vi "DriveBegin.vi"(8 "error in (no error)":errorcluster) -> (0 "error out":errorcluster)   [LabVIEW 2020]
doc: "Begin for Drive\n\nInputs:\n -- Error in -- Error cluster -- propagated error input\n\nOutputs:\n -- Error out -- Error cluster -- progated error output"
uses:
  <vilib>/Rock Robotics/SystemInterfaces/DIO/FPGA_DIOPWMChannel.ctl
  DriveGlobal.vi
  <vilib>/Rock Robotics/WPI/ThirdParty/JAS_Junk/TrajLib/Trajectory_Library.lvlib
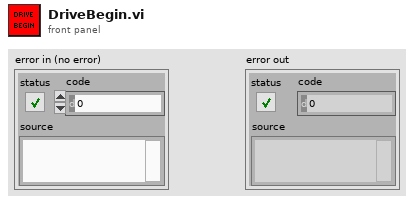
[diagram p1: front panel]
types:
  T1 = typedef "FPGA_DIOPWMChannel.ctl" = enum8{"PWM 0", "PWM 1", "PWM 2", "PWM 3", "PWM 4", "PWM 5", "PWM 6", "PWM 7", "PWM 8", "PWM 9", "PWM MXP 0", "PWM MXP 1", "PWM MXP 2", "PWM MXP 3", "PWM MXP 4", "PWM MXP 5", "PWM MXP 6", "PWM MXP 7", "PWM MXP 8", "PWM MXP 9", "Invalid"}
  T2 = typedef "Trajectory_Library.lvlib/TRANSLATION2D.ctl" = cluster{"X":dbl, "Y":dbl}
  T3 = typedef "Trajectory_Library.lvlib/SWERVE_DRIVE_KINEMATICS.ctl" = cluster{"NumModules":i32, "InverseKinematics":T4, "ForwardKinematics":T4, "Modules":T2[], "PrevCoR":T2, "SavedModuleStates":T5[]}
  T4 = typedef "NI_Matrix.lvlib/RealMatrix.ctl" = dbl[][]
  T5 = typedef "Trajectory_Library.lvlib/SWERVE_DRIVE_MODULE_STATE.ctl" = cluster{"Speed":dbl, "Angle":T6}
  T6 = typedef "Trajectory_Library.lvlib/ROTATION2D.ctl" = cluster{"VALUE":dbl, "COS":dbl, "SIN":dbl}
  T7 = typedef "WPI_PWMDeviceRef.ctl" = cluster{"DeviceStatus":errorcluster, "PWM Channel":T1}
  T8 = typedef "ADIS16470 Device Reference.ctl" = cluster{"DevStatus":errorcluster, "Hardware Config":T9, "Calibration Complete":refnum<notifier>, "Status Reference":refnum<data-value>, "Data Reference":refnum<data-value>, "Sychronous Process VI":T13, "Cmd FIFO":refnum<k33>, "Source":T14, "Data FIFO":refnum<k33>, "Calibration Time (ms)":u32, "Data Reference":refnum<data-value>}
  T9 = typedef "ADIS16470 Hardware Configuration.ctl" = cluster{"SPI Clock Rate (Hz)":dbl, "IMU SPI Mode (3)":T10, "IMU Reset Pin":T11, "IMU SPI Bus":T12, "IMU Data Ready Pin":T11, "Stall Config":cluster{"Pow2BytesPerRead":u8, "StallTicks":u16, "CsToSclkTicks":u8}}
  T10 = typedef "WPI_SPIMode.ctl" = enum16{"Mode 0 (Clk Idle Low,Sample on Leading)", "Mode 1 (Clk Idle Low,Sample on Trailing)", "Mode 2 (Clk Idle High,Sample on Leading)", "Mode 3 (Clk Idle High,Sample on Trailing)"}
  T11 = typedef "FPGA_DIOChannel.ctl" = enum8{"DIO 0", "DIO 1", "DIO 2", "DIO 3", "DIO 4", "DIO 5", "DIO 6", "DIO 7", "DIO 8", "DIO 9", "DIO MXP 0", "DIO MXP 1", "DIO MXP 2", "DIO MXP 3", "DIO MXP 4", "DIO MXP 5", "DIO MXP 6", "DIO MXP 7", "DIO MXP 8", "DIO MXP 9", "DIO MXP 10", "DIO MXP 11", "DIO MXP 12", "DIO MXP 13", "DIO MXP 14", "DIO MXP 15", "SPI Port CS1", "SPI Port CS2", "SPI Port CS3", "SPI Port MISO", "SPI Port MOSI", "Invalid"}
  T12 = typedef "spi_bus.ctl" = enum16{"SPI On-Board, CS0", "SPI On-Board, CS1", "SPI On-Board, CS2", "SPI On-Board, CS3", "SPI MXP", "Invalid"}
  T13 = typedef "ADIS16470 Process.ctl" = refnum<vi>
  T14 = typedef "FPGA_CounterEncoderSourceConvertionLVSourceType.ctl" = cluster{"DevStatus":errorcluster, "AnalogTriggerMode?":bool, "DigitalMode":cluster{"DIO Channel":T15}, "AnalogTriggerMode":cluster{"AnalogTriggerIndex":T16, "OutputType":T17}}
  T15 = typedef "FPGA_DIODigitalSourceChannel.ctl" = enum8{"DIO 0", "DIO 1", "DIO 2", "DIO 3", "DIO 4", "DIO 5", "DIO 6", "DIO 7", "DIO 8", "DIO 9", "DIO MXP 0", "DIO MXP 1", "DIO MXP 2", "DIO MXP 3", "DIO MXP 4", "DIO MXP 5", "DIO MXP 6", "DIO MXP 7", "DIO MXP 8", "DIO MXP 9", "DIO MXP 10", "DIO MXP 11", "DIO MXP 12", "DIO MXP 13", "DIO MXP 14", "DIO MXP 15", "SPI Port CS1", "SPI Port CS2", "SPI Port CS3", "SPI Port MISO", "SPI Port MOSI", "Disabled"}
  T16 = typedef "FPGA_AnalogTriggerIndex.ctl" = enum8{"Trig 0", "Trig 1", "Trig 2", "Trig 3", "Trig 4", "Trig 5", "Trig 6", "Trig 7", "Invalid"}
  T17 = typedef "FPGA_AnalogTriggerOutType.ctl" = enum16{"InWindow", "TriggerState", "Rising", "Falling"}
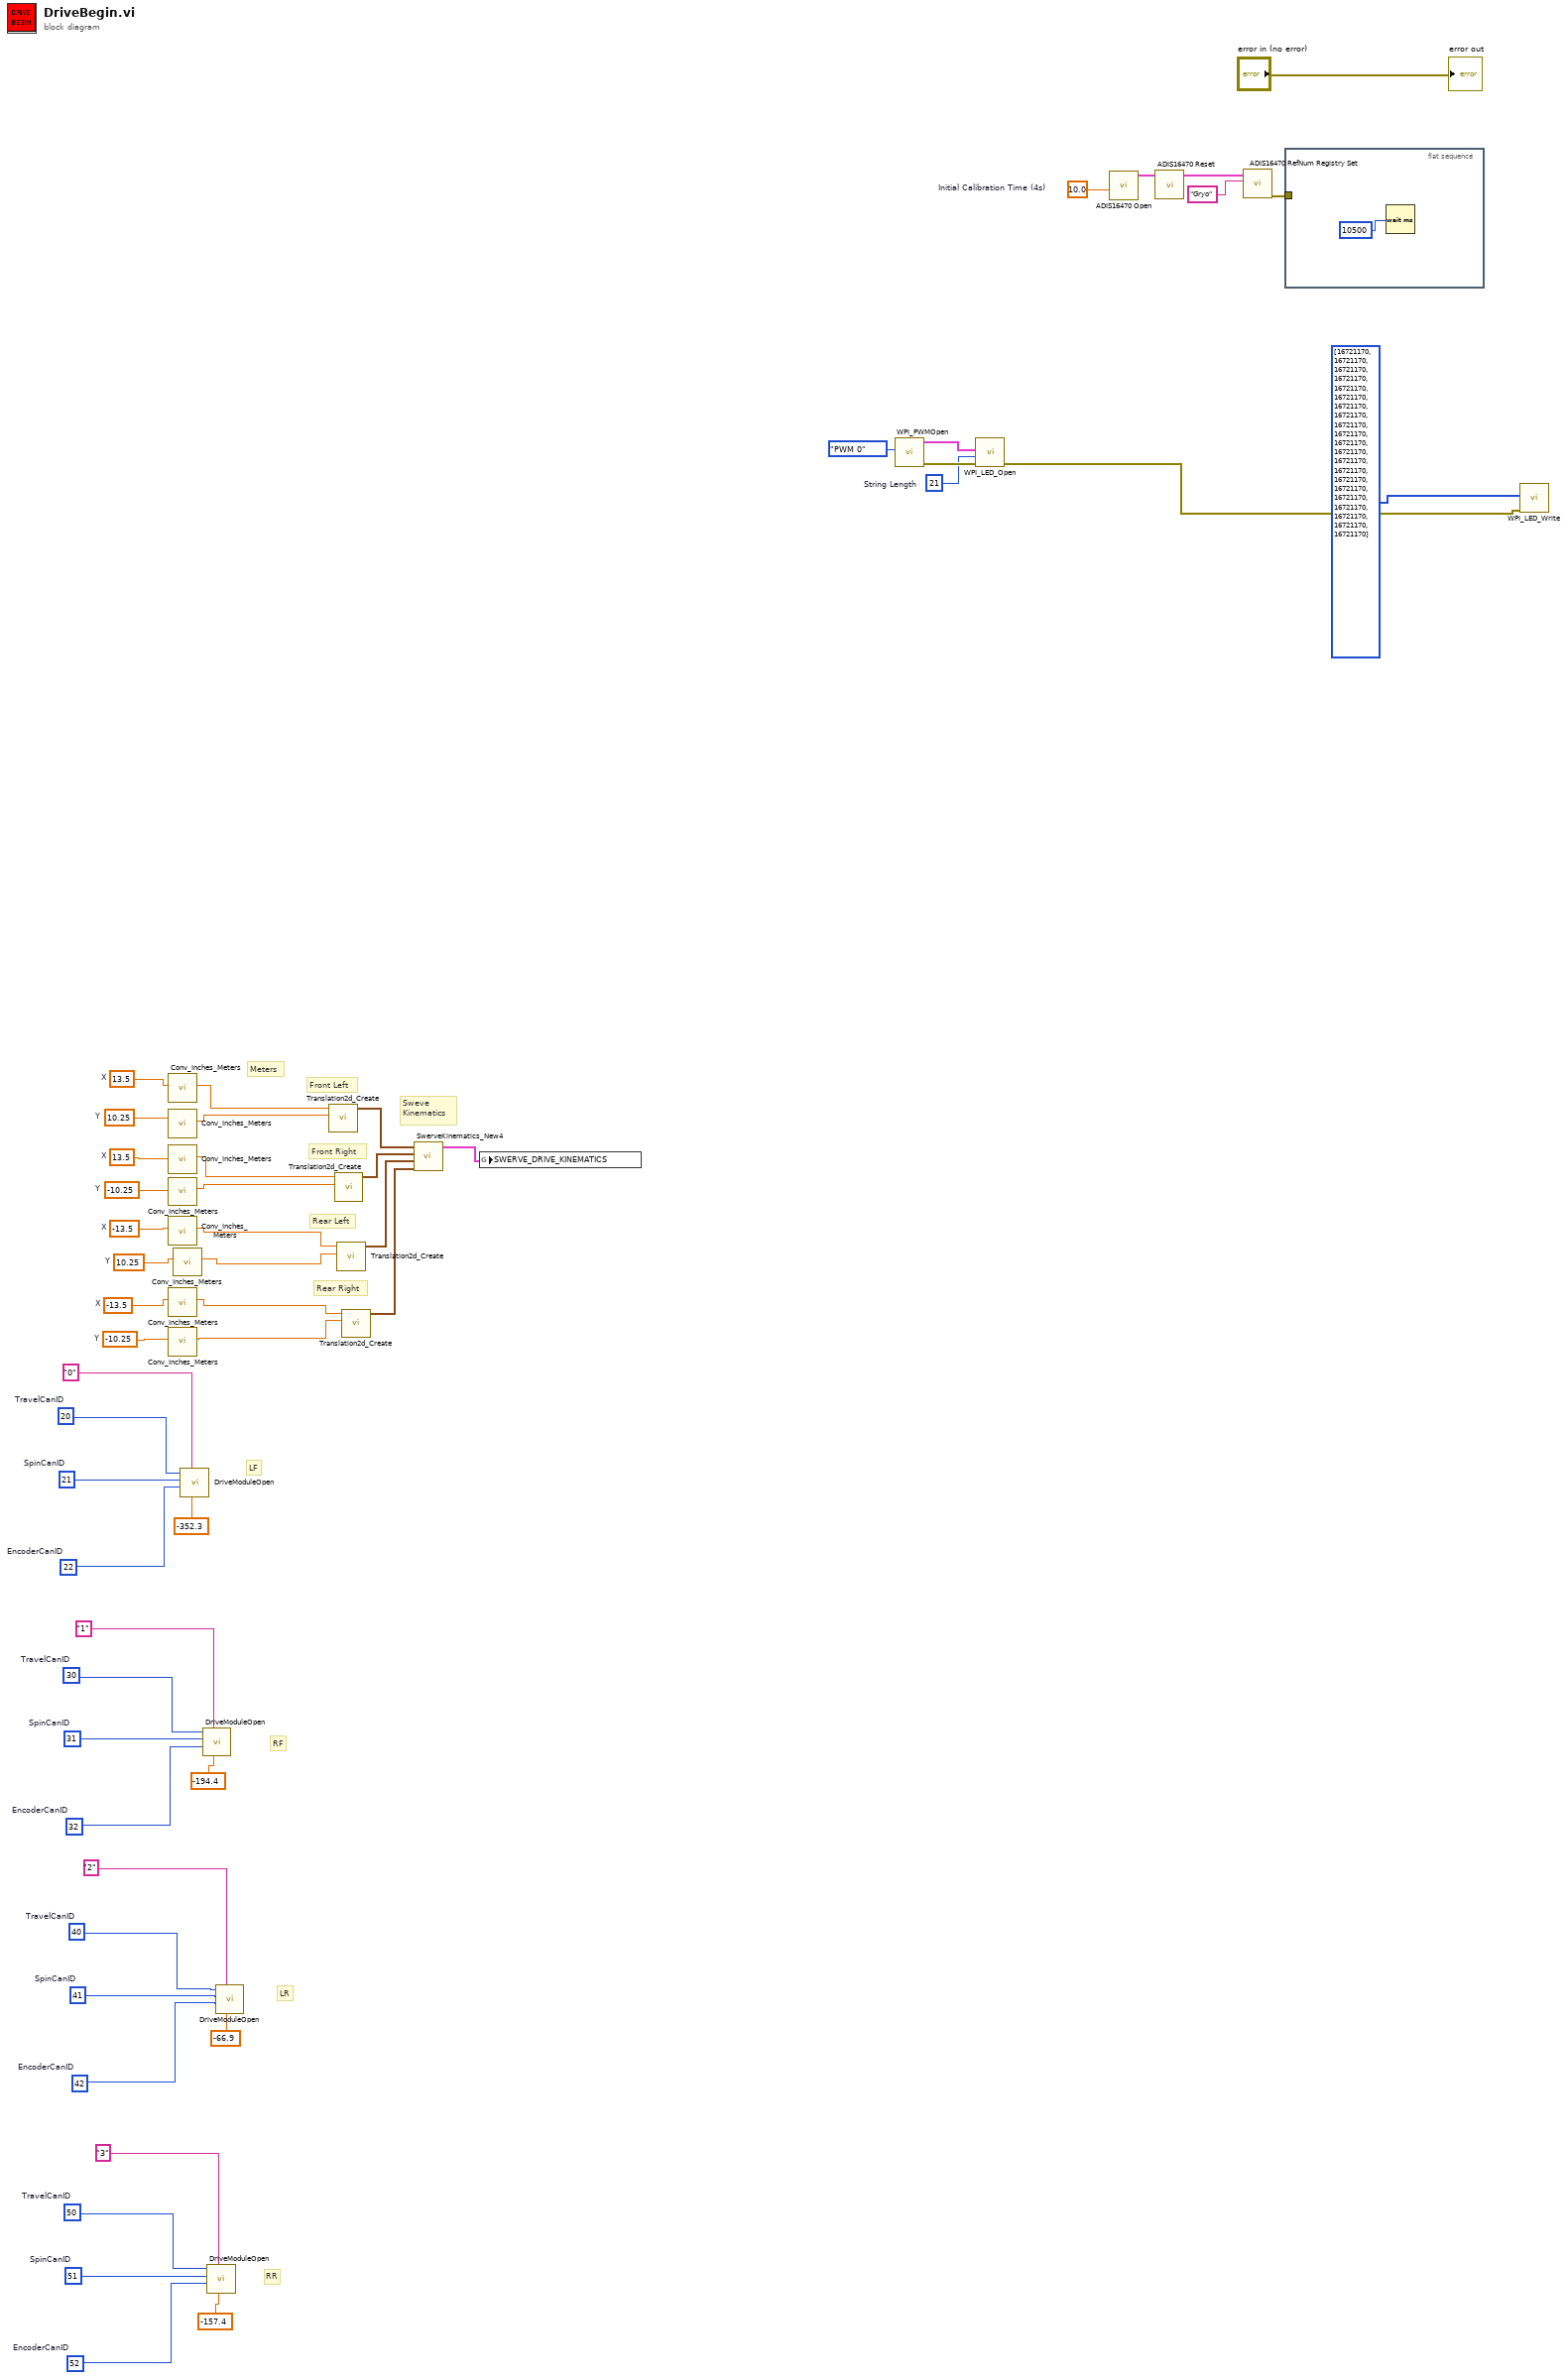
[diagram p0: block diagram]
diagram:
  w7 = u8 50  # TravelCanID
  w6 = u8 51  # SpinCanID
  w5 = u8 52  # EncoderCanID
  w10 = u8 40  # TravelCanID
  w9 = u8 41  # SpinCanID
  w8 = u8 42  # EncoderCanID
  w13 = u8 30  # TravelCanID
  w12 = u8 31  # SpinCanID
  w11 = u8 32  # EncoderCanID
  w14 = u8 20  # TravelCanID
  w15 = u8 21  # SpinCanID
  w16 = u8 22  # EncoderCanID
  w23 = -13.5  # X
  w22 = -10.25  # Y
  w25 = -13.5  # X
  w24 = 10.25  # Y
  w27 = 13.5  # X
  w26 = -10.25  # Y
  w29 = 13.5  # X
  w28 = 10.25  # Y
  w45 = u16 21  # String Length
  w51 = 10.0  # Initial Calibration Time (4s)
  # "RR"
  # "LR"
  # "RF"
  # "LF"
  # "Meters"
  # "Sweve\nKinematics"
  # "Rear Right"
  # "Rear Left"
  # "Front Right"
  # "Front Left"
  n1 = call <vilib>:"Conv_Inches_Meters.vi"("INCH"=w29) -> ("Meters"=w30:dbl)  [unwired: 10 in]
  n2 = call <vilib>:"Conv_Inches_Meters.vi"("INCH"=w28) -> ("Meters"=w31:dbl)  [unwired: 10 in]
  n3 = call <vilib>:"Conv_Inches_Meters.vi"("INCH"=w27) -> ("Meters"=w32:dbl)  [unwired: 10 in]
  n4 = call <vilib>:"Conv_Inches_Meters.vi"("INCH"=w26) -> ("Meters"=w33:dbl)  [unwired: 10 in]
  n5 = call <vilib>:"Conv_Inches_Meters.vi"("INCH"=w25) -> ("Meters"=w34:dbl)  [unwired: 10 in]
  n6 = call <vilib>:"Conv_Inches_Meters.vi"("INCH"=w23) -> ("Meters"=w37:dbl)  [unwired: 10 in]
  n7 = call <vilib>:"Conv_Inches_Meters.vi"("INCH"=w22) -> ("Meters"=w36:dbl)  [unwired: 10 in]
  n8 = call <vilib>:"Conv_Inches_Meters.vi"("INCH"=w24) -> ("Meters"=w35:dbl)  [unwired: 10 in]
  n9 = call "DriveModuleOpen.vi"("Magnet Offset (Degrees)"=-352.3, "ModualNamePrefix"="0", "EncoderCanID"=w16, "SpinCanID"=w15, "TravelCanID"=w14) -> ()  [unwired: 6 in, 1 out]
  n10 = call "DriveModuleOpen.vi"("Magnet Offset (Degrees)"=-194.4, "ModualNamePrefix"="1", "EncoderCanID"=w11, "SpinCanID"=w12, "TravelCanID"=w13) -> ()  [unwired: 6 in, 1 out]
  n11 = call "DriveModuleOpen.vi"("Magnet Offset (Degrees)"=-157.4, "ModualNamePrefix"="3", "EncoderCanID"=w5, "SpinCanID"=w6, "TravelCanID"=w7) -> ()  [unwired: 6 in, 1 out]
  n12 = call "DriveModuleOpen.vi"("Magnet Offset (Degrees)"=-66.9, "ModualNamePrefix"="2", "EncoderCanID"=w8, "SpinCanID"=w9, "TravelCanID"=w10) -> ()  [unwired: 6 in, 1 out]
  n13 = call <vilib>:"Translation2d_Create.vi"("Y"=w31, "X"=w30) -> ("TRANSLATION"=w38:T2)  [unwired: 9 in]
  n14 = call <vilib>:"Translation2d_Create.vi"("Y"=w33, "X"=w32) -> ("TRANSLATION"=w39:T2)  [unwired: 9 in]
  n15 = call <vilib>:"Translation2d_Create.vi"("Y"=w35, "X"=w34) -> ("TRANSLATION"=w40:T2)  [unwired: 9 in]
  n16 = call <vilib>:"Translation2d_Create.vi"("Y"=w36, "X"=w37) -> ("TRANSLATION"=w41:T2)  [unwired: 9 in]
  n17 = call <vilib>:"SwerveKinematics_New4.vi"("wheel 3"=w41, "wheel 2"=w40, "wheel 1"=w39, "wheel 0"=w38) -> ("SWERVE_DRIVE_KINEMATICS"=w21:T3)  [unwired: 7 in]
  n18 = global write "DriveGlobal.vi" "SWERVE_DRIVE_KINEMATICS"(w21) -> ()
  n19 = call <vilib>:"WPI_PWMOpen.vi"("PWM Channel"=FPGA_DIOPWMChannel."PWM 0") -> ("error out"=w46:errorcluster, "PWMDeviceRef"=w47:T7)  [unwired: 9 in]
  n20 = call <vilib>:"WPI_LED_Open.vi"("error in"=w46, "String Length"=w45, "PWMDeviceRef"=w47) -> ("error out"=w42:errorcluster)  [unwired: 8 in]
  n21 = call <vilib>:"ADIS16470 Open.vi"("Initial Calibration Time (4s)"=w51) -> ("ADIS16470DevRef"=w50:T8)  [unwired: 9 in, 1 out]
  n22 = call <vilib>:"ADIS16470 Reset.vi"("ADIS16470DevRef"=w50) -> ("ADIS16470DevRef"=w49:T8)  [unwired: 9 in, 1 out]
  n23 = call <vilib>:"ADIS16470 RefNum Registry Set.vi"("refnum name"="Gryo", "ADIS16470DevRef in"=w49) -> ("error out"=w48:errorcluster)  [unwired: 8 in, 1 out]
  n24 = flat-sequence {
    tunnel: w48 -> [_]
    frame #0 {
      n25 = Wait (ms)(milliseconds to wait=u32 10500) -> ()  [unwired: 1 out]
    }
  }
  n26 = call <vilib>:"WPI_LED_Write.vi"("error in"=w42, "Color Array"=u32[] [16721170, 16721170, 16721170, 16721170, 16721170, 16721170, 16721170, 16721170, 16721170, 16721170, 16721170, 16721170, 16721170, 16721170, 16721170, 16721170, 16721170, 16721170, 16721170, 16721170, 16721170]) -> ()  [unwired: 9 in, 1 out]
  "error out" <- "error in (no error)"
